vi "Hardware-Phase2SensorsSetupCalPoints.vi"(10 "UEGO2 Disable":bool, 11 "UEGO1 Disable":bool) -> (0 "VR Hall Clear Faults":bool, 1 "SensorControl":T2={"UEGO1Enable"=FALSE, "UEGO2Enable"=FALSE, "UEGO1Range"=FALSE, "UEGO2Range"=FALSE, "FilterCutoff (Hz)"=10.0}, 2 "VR-Hall Arming/Threshold [V]":dbl[](array[numeric]), 3 "VR-Hall Mode Select":T1[](array[typedef])=[enum."VR Adaptive Arm", enum."VR Adaptive Arm", enum."VR Adaptive Arm", enum."VR Adaptive Arm", enum."VR Adaptive Arm"])   [LabVIEW 2016, in "DSI-RT.lvlib"]
uses:
  DSI-RT.lvlib
  <vilib>/Powertrain Controls/Device Drivers/VR-Hall/RevC/Real-Time/Support/Vr_Hall_mode_control_revc.ctl
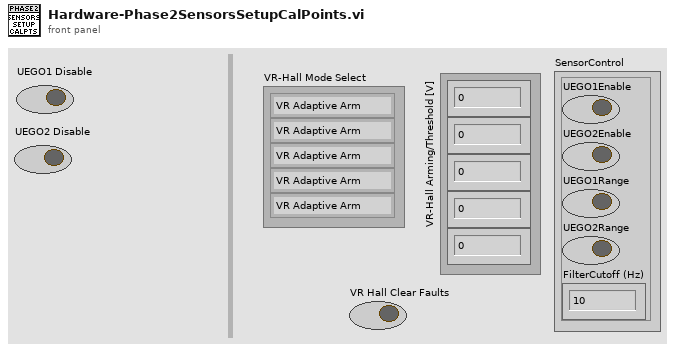
[diagram p1: front panel]
types:
  T1 = typedef "Vr_Hall_mode_control_revc.ctl" = enum32{"VR Adaptive Arm", "VR Manual Arm", "Hall", "Hall w/ Pull-up"}
  T2 = cluster{"UEGO1Enable":bool, "UEGO2Enable":bool, "UEGO1Range":bool, "UEGO2Range":bool, "FilterCutoff (Hz)":dbl}
  T3 = cluster{bool, bool, "Value":bool, "Value":bool, "Value":sgl}
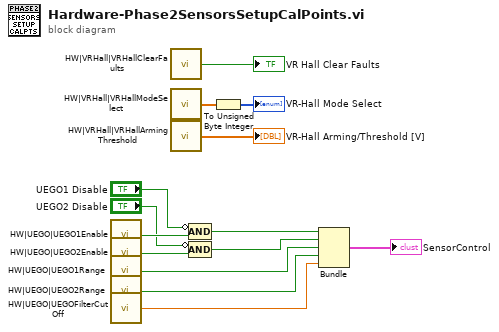
[diagram p0: block diagram]
diagram:
  n1 = call "HW|UEGO|UEGO1Enable"() -> ("Value"=w6:bool)
  n2 = call "HW|UEGO|UEGO2Enable"() -> ("Value"=w2:bool)
  n3 = call "HW|UEGO|UEGO1Range"() -> ("Value"=w12:bool)
  n4 = call "HW|UEGO|UEGO2Range"() -> ("Value"=w11:bool)
  n5 = call "HW|UEGO|UEGOFilterCutOff"() -> ("Value"=w10:sgl)
  n6 = call "HW|VRHall|VRHallClearFaults"() -> ("Value"=→"VR Hall Clear Faults":bool)
  n7 = call "HW|VRHall|VRHallModeSelect"() -> ("Value"=w14:sgl[])
  n8 = call "HW|VRHall|VRHallArmingThreshold"() -> ("Value"=→"VR-Hall Arming/Threshold [V]":sgl[])
  n9 = Compound Arithmetic op=AND(invert "UEGO1 Disable", w6) -> (w5:bool)
  n10 = Compound Arithmetic op=AND(invert "UEGO2 Disable", w2) -> (w4:bool)
  n11 = To Unsigned Byte Integer(number=w14) -> (unsigned 8bit integer=→"VR-Hall Mode Select":u8[])
  n12 = Bundle(w5, w4, "Value"=w12, "Value"=w11, "Value"=w10) -> (→"SensorControl":T3)  [unwired: 1 in]
